vi "CMN_SetBuffers.vi"(9 "deftransferbufsize":u32=131072, 10 "BuffersDimensions":T1, 11 "database name":string="DBS") -> ()   [LabVIEW 2016]
uses:
  CMN_Buffers.ctl
  DBSHAND/private/vis/DatabaseHand_Element_Set(U32).vi
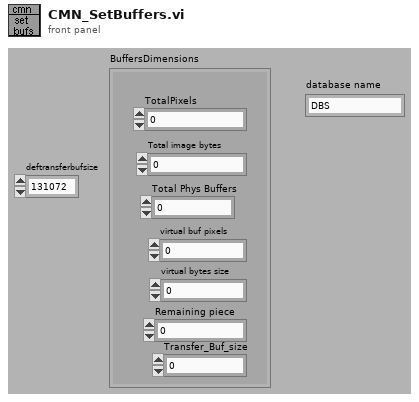
[diagram p1: front panel]
types:
  T1 = typedef "CMN_Buffers.ctl" = cluster{"TotalPixels":u32, "Total image bytes":u32, "Total Phys Buffers":u32, "virtual buf pixels":u32, "virtual bytes size":u32, "Remaining piece":u32, "Transfer_Buf_size":u32}
  T2 = typedef "DatabaseHand_RefNum.ctl" = refnum<vi>
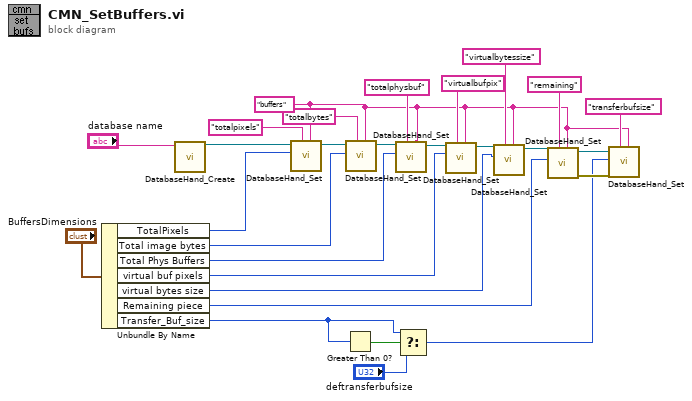
[diagram p0: block diagram]
diagram:
  w1 = "buffers" ("group")
  n1 = Unbundle By Name("BuffersDimensions") -> ("TotalPixels"=w14:u32, "Total image bytes"=w13:u32, "Total Phys Buffers"=w12:u32, "virtual buf pixels"=w11:u32, "virtual bytes size"=w10:u32, "Remaining piece"=w9:u32, "Transfer_Buf_size"=w4:u32)
  n2 = call "DatabaseHand_Create.vi"("Name"="database name") -> ("Database RefNum out"=w27:T2)  [unwired: 1 in, 9 out]
  n3 = call-poly "DatabaseHand_Set.vi"("group"=w1, "name"="totalpixels", "value"=w14, "Database RefNum in"=w27) -> ("Database RefNum out"=w26:T2)  [unwired: 4 in, 3 out]
  n4 = Greater Than 0?(x=w4) -> (x > 0?=w5:bool)
  n5 = call-poly "DatabaseHand_Set.vi"("group"=w1, "name"="totalbytes", "value"=w13, "Database RefNum in"=w26) -> ("Database RefNum out"=w25:T2)  [unwired: 4 in, 3 out]
  n6 = call-poly "DatabaseHand_Set.vi"("group"=w1, "name"="totalphysbuf", "value"=w12, "Database RefNum in"=w25) -> ("Database RefNum out"=w24:T2)  [unwired: 4 in, 3 out]
  n7 = Select(t=w4, s=w5, f="deftransferbufsize") -> (s? t:f=w2:u32)
  n8 = call-poly "DatabaseHand_Set.vi"("group"=w1, "name"="virtualbufpix", "value"=w11, "Database RefNum in"=w24) -> ("Database RefNum out"=w23:T2)  [unwired: 4 in, 3 out]
  n9 = call-poly "DatabaseHand_Set.vi"("group"=w1, "name"="virtualbytessize", "value"=w10, "Database RefNum in"=w23) -> ("Database RefNum out"=w22:T2)  [unwired: 4 in, 3 out]
  n10 = call-poly "DatabaseHand_Set.vi"("group"=w1, "name"="remaining", "value"=w9, "Database RefNum in"=w22) -> ("error out"=w7:errorcluster, "Database RefNum out"=w8:T2)  [unwired: 4 in, 2 out]
  n11 = call-poly "DatabaseHand_Set.vi"("group"=w1, "name"="transferbufsize", "error in (no error)"=w7, "value"=w2, "Database RefNum in"=w8) -> ()  [unwired: 3 in, 4 out]
